vi "Global.vi"() -> ()   [LabVIEW 2016]
panel:
  in  "手腕平滑时间":u32=10
  in  "小手指平滑时间":u32=35
  in  "手腕当前值":u8=180
  in  "小手指当前值":u8=116
  in  "无名指平滑时间":u32=10
  in  "中指平滑时间":u32=35
  in  "无名指当前值":u8=52
  in  "中指当前值":u8=135
  in  "食指平滑时间":u32=10
  in  "拇指平滑时间":u32=35
  in  "食指当前值":u8=42
  in  "拇指当前值":u8=136
  in  "转台平滑时间":u32=10
  in  "手臂平滑时间":u32=35
  in  "转台当前值":u8=180
  in  "手臂当前值":u8=84
  in  "手指参数":T1={" 拇指最大值"=136.0, " 拇指最小值"=72.0, "食指最大值"=146.0, " 中指最大值"=135.0, " 无名指最大值"=143.0, "食指最小值"=42.0, " 中指最小值"=37.0, " 无名指最小值"=52.0, "小手指最小值"=36.0, " 小手指最大值"=116.0, "手腕最大值"=180.0, "手腕最小值"=0.0, "手臂最小值 "=15.0, "手臂最大值 "=84.0, "转台最小值 "=26.0, "转台最大值"=180.0}
  out "在线测试数据清空":bool
  in  "StopNum":bool[](array[boolean])
  out "角度 主面板":dbl
  in  "密   码：":string="7872105"
  in  "用户名：":string="俞忠达"
  out "级别":u16(ring)=1 items=["其他", "普通用户", "管理员"]
  in  "停止位":u16(ring)=10 items=["1.0"=10, "1.5"=15, "2.0"=20]
  out "数据位":u16=8 min=5 max=8 step=1
  out "波特率":u32=115200
  in  "串口":refnum<visa-resource-name>="COM3"
  out "串口状态":bool
  out "在线测试数据":string[][](array[string])=[["30", "2015/12/2 18:50:33", "俞忠达", "JMS", "0", "8", "-2.24"]]
  in  "Grade":string(combo)="Admin"
  in  "型号":string="J01"
  out "个数":dbl
  out "级数":dbl
  out "角度":dbl
  out "个数状态":bool
  out "级数状态":bool
  out "角度状态":bool
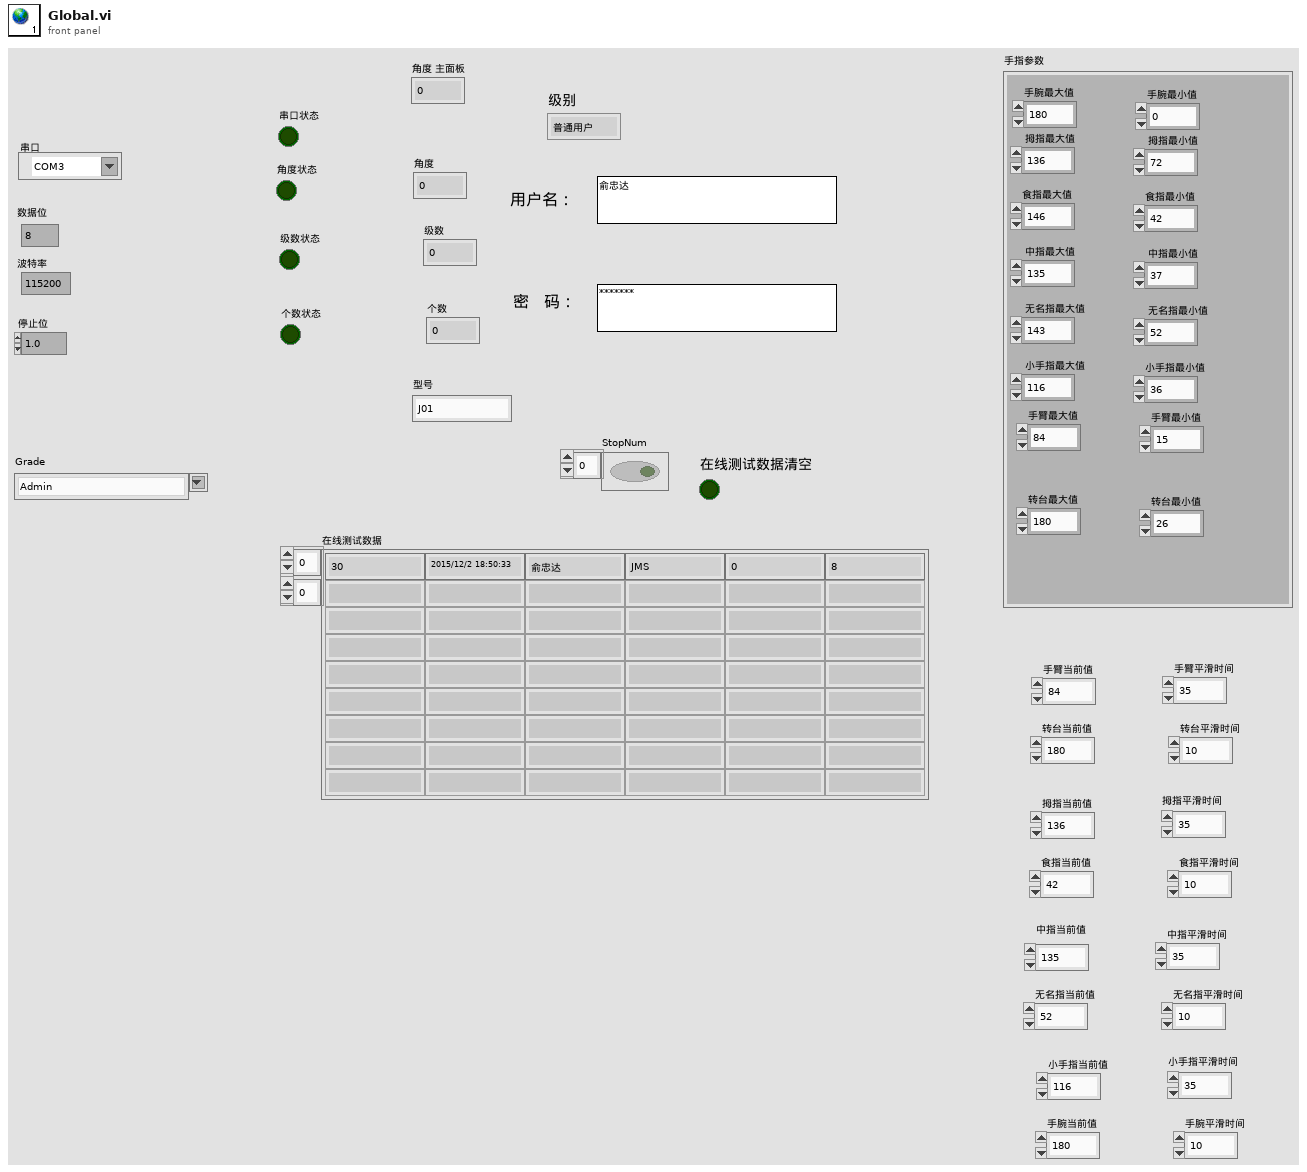
[diagram p1: front panel]
types:
  T1 = cluster{" 拇指最大值":dbl, " 拇指最小值":dbl, "食指最大值":dbl, " 中指最大值":dbl, " 无名指最大值":dbl, "食指最小值":dbl, " 中指最小值":dbl, " 无名指最小值":dbl, "小手指最小值":dbl, " 小手指最大值":dbl, "手腕最大值":dbl, "手腕最小值":dbl, "手臂最小值 ":dbl, "手臂最大值 ":dbl, "转台最小值 ":dbl, "转台最大值":dbl}
diagram:
